vi "自动载入减计数器.vi"(8 "error in":errorcluster, 9 "preset value":u32=10, 10 "load":bool, 11 "count down":bool) -> (0 "error out":errorcluster, 1 "counter value":u32, 3 "done":bool)   [LabVIEW 2012]
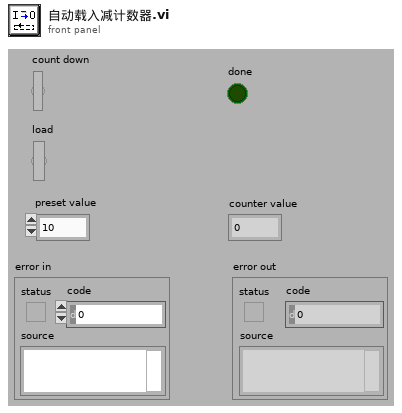
[diagram p1: front panel]
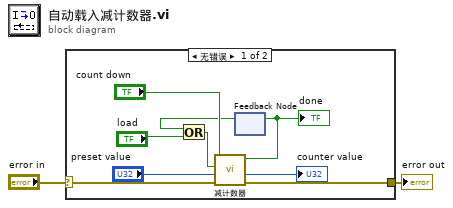
[diagram p0: block diagram]
diagram:
  n1 = case shown="无错误" "error in" {
    selector: "error in" -> [w11 w12]
    tunnel: [w10 w12] -> w2
    frame No Error {
      n2 = feedback #1() -> (w4:bool)  [unwired: 1 in]
      n3 = Or(x=w4, y="load") -> (x .or. y?=w3:bool)
      n4 = call "减计数器.vi"("error in"=w11, "preset value"="preset value", "load"=w3, "count down"="count down") -> ("error out"=w10:errorcluster, "counter value"=→"counter value":u32, "done"=w6:bool)  [unwired: 5 in]
      "done" <- w6
      n5 = feedback-in #1(w6) -> ()
    }
    frame Error {
    }
  }
  "error out" <- w2
